vi "Cannon camera offset.vi"(1 "Offset (from center axis to camera lens)":dbl, 2 "Distance (from camera)":dbl, 3 "Camera angle":dbl) -> (0 "Distance from cannon":dbl)   [LabVIEW 2012]
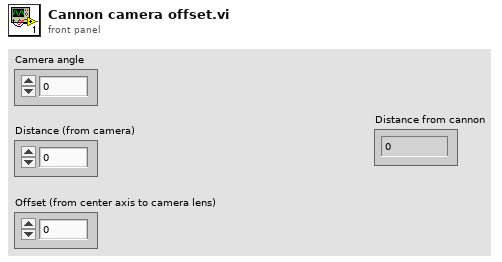
[diagram p1: front panel]
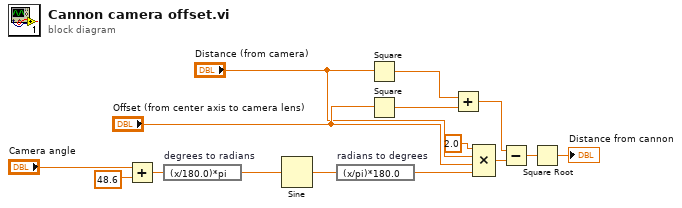
[diagram p0: block diagram]
diagram:
  n1 = Add(x="Camera angle", y=48.6) -> (x+y=w3:dbl)
  n2 = expression code="(x/180.0)*pi" "degrees to radians"(w3) -> (w8:dbl)
  n3 = Sine(x=w8) -> (sin(x)=w7:dbl)
  n4 = expression code="(x/pi)*180.0" "radians to degrees"(w7) -> (w6:dbl)
  n5 = Square(x="Distance (from camera)") -> (x^2=w11:dbl)
  n6 = Square(x="Offset (from center axis to camera lens)") -> (x^2=w15:dbl)
  n7 = Add(x=w11, y=w15) -> (x+y=w14:dbl)
  n8 = Compound Arithmetic op=MULTIPLY(2.0 ("value"), "Distance (from camera)", "Offset (from center axis to camera lens)", w6) -> (w13:dbl)
  n9 = Subtract(x=w14, y=w13) -> (x-y=w2:dbl)
  n10 = Square Root(x=w2) -> (sqrt(x)=→"Distance from cannon":dbl)
